vi "FTW-SQLite-RandomBLOB.vi"(0 "Number of Bytes":i32=1024, 11 "error in":errorcluster) -> (4 "Random BLOB":string, 15 "error out":errorcluster)   [LabVIEW 2013, in "FTW-SQLite-Connector.lvclass"]
uses:
  FTW-SQLite-Connector.lvclass
panel:
  # "Inputs"
  # "Outputs"
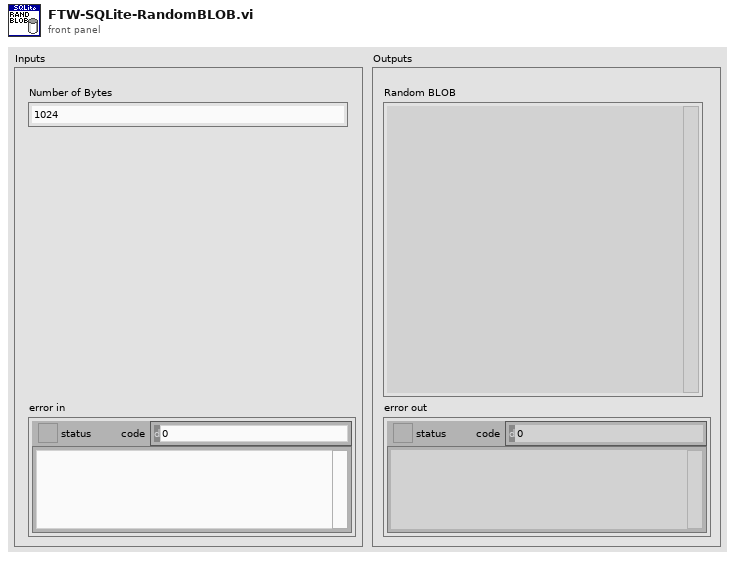
[diagram p1: front panel]
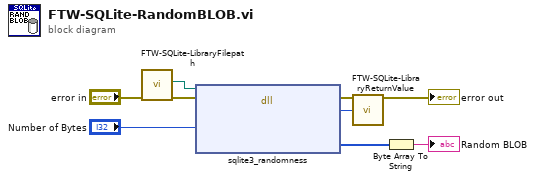
[diagram p0: block diagram]
diagram:
  n1 = call "FTW-SQLite-LibraryFilepath.vi"("error in"="error in") -> ("error out"=w9:errorcluster, "SQLite Library Filepath"=w8:path)  [unwired: 8 in, 1 out]
  n2 = dll-call lib="?" fn="sqlite3_randomness"(path in=w8, error in=w9, "Number of Bytes"="Number of Bytes") -> (error out=w6:errorcluster, "Return Value"=w4:i32, "Random Bytes Buffer"=w2:u8[])  [unwired: 3 in, 1 out]
  n3 = call "FTW-SQLite-LibraryReturnValue.vi"("error in"=w6, "Return Value"=w4) -> ("error out"=→"error out":errorcluster)  [unwired: 13 in]
  n4 = Byte Array To String(unsigned byte array=w2) -> (string=→"Random BLOB":string)
